vi "Maestro Ethernet Communication Example V1.00.00.vi"() -> ()   [LabVIEW 2021]
doc: "Data Client.vi displays data sent via TCP from Data Server. Once a TCP connection is open, the VI reads 4 bytes to determine the amount of data being sent. It then reads and charts that many bytes. If an error occurs or the stop button is pressed, it sends a \"Q\" to the Data Sender to notify it to quit."
panel:
  in  "file path":path
  in  "Save":bool
  in  "Connect":bool
  out "Readings":dbl format="%.6e"
  out "Maestro Online":bool
  in  "Send":bool
  in  "Command":string="*CAU"
  out "Waveform Chart":dbl(graph)=2.12187e-08
  out "Response":string="\r\n"
  in  "stop":bool
  in  "Address":string="192.168.0.44"
  in  "Port":i16=5000 min=1025 step=1
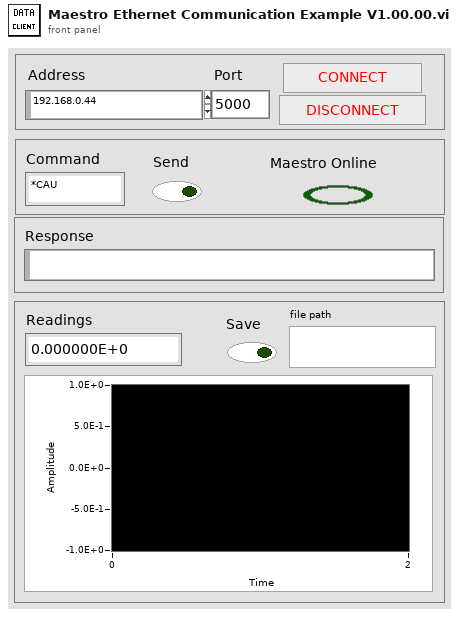
[diagram p1: front panel]
types:
  T1 = enum16{"Standard", "Buffered", "CRLF", "Immediate"}
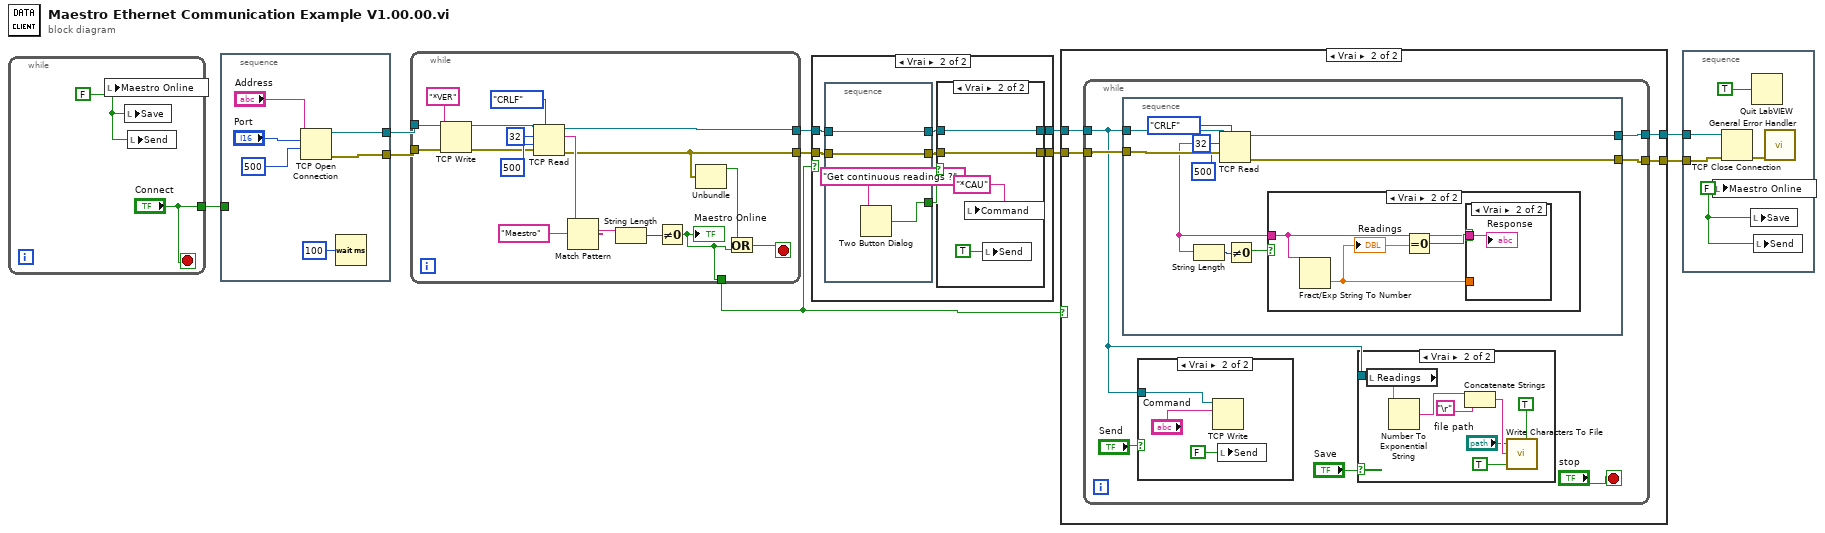
[diagram p0: block diagram]
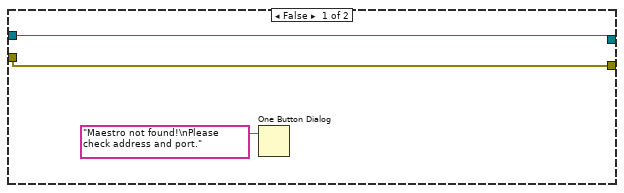
[diagram p4: hidden frame]
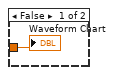
[diagram p7: hidden frame]
diagram:
  n1 = while {
    tunnel: ["Connect"] -> w2
    stop <- "Connect" stop-if-true
    w11 = FALSE ("Reception")
    n2 = local write "Maestro Online"(w11) -> ()
    n3 = local write "Save"(w11) -> ()
    n4 = local write "Send"(w11) -> ()
  }
  n5 = stacked-sequence {
    tunnel: [w16] -> w8
    tunnel: [w15] -> w7
    tunnel: w2 -> [_]
    frame #0 {
      n6 = TCP Open Connection(address="Address", remote port or service name="Port", timeout ms (60000)=500) -> (connection ID=w16:refnum<k5>, error out=w15:errorcluster)  [unwired: 2 in]
      n7 = Wait (ms)(milliseconds to wait=u32 100) -> ()  [unwired: 1 out]
    }
  }
  n8 = while {
    tunnel: [w35] -> w3
    tunnel: [w21] -> w4
    tunnel: w8 -> [w34]
    tunnel: w7 -> [w33]
    tunnel: [w19] -> w1
    stop <- w20 stop-if-true
    n9 = TCP Write(connection ID=w34, data in="*VER" ("string"), error in (no error)=w33) -> (connection ID out=w24:refnum<k5>, error out=w23:errorcluster)  [unwired: 1 in, 1 out]
    n10 = TCP Read(connection ID=w24, bytes to read=32, error in (no error)=w23, 7:T1."CRLF" ("mode (standard)"), 9:500 ("timeout ms (25000)")) -> (connection ID out=w35:refnum<k5>, data out=w29:string, error out=w21:errorcluster)
    n11 = Match Pattern(string=w29, regular expression="Maestro") -> (match substring=w26:string)  [unwired: 1 in, 3 out]
    n12 = String Length(string=w26) -> (length=w27:i32)
    n13 = Not Equal To 0?(x=w27) -> (x != 0?=w19:bool)
    "Maestro Online" <- w19
    n14 = Unbundle(w21) -> ("status"=w22:bool)  [unwired: 2 out]
    n15 = Or(x=w22, y=w19) -> (x .or. y?=w20:bool)
  }
  n16 = case shown="Vrai" w1 {
    tunnel: [w37 w44] -> w6
    tunnel: [w36 w43] -> w5
    tunnel: w4 -> [w37 w41]
    tunnel: w3 -> [w36 w40]
    frame False {
    }
    frame True {
      n17 = stacked-sequence {
        tunnel: [w48] -> w42
        tunnel: w41 -> [w47]
        tunnel: w40 -> [w46]
        tunnel: [w47] -> w39
        tunnel: [w46] -> w38
        frame #0 {
          n18 = Two Button Dialog(message="Get continuous readings ?") -> (T button?=w48:bool)  [unwired: 2 in]
        }
      }
      n19 = case shown="Vrai" w42 {
        tunnel: w39 -> [w49 w54]
        tunnel: [w49 w54] -> w44
        tunnel: [w50 w53] -> w43
        tunnel: w38 -> [w50 w53]
        frame False {
        }
        frame True {
          n20 = local write "Command"("*CAU" ("string")) -> ()
          n21 = local write "Send"(TRUE ("Send")) -> ()
        }
      }
    }
  }
  n22 = case shown="Vrai" w1 {
    tunnel: w5 -> [w57 w61]
    tunnel: w6 -> [w56 w60]
    tunnel: [w56 w59] -> w10
    tunnel: [w57 w58] -> w9
    frame False {
      n23 = One Button Dialog(message="Maestro not found!\nPlease check address and port.") -> ()  [unwired: 1 in, 1 out]
    }
    frame True {
      n24 = while {
        tunnel: w60 -> [w67]
        tunnel: w61 -> [w62]
        tunnel: [w66] -> w59
        tunnel: [w65] -> w58
        stop <- "stop" stop-if-true
        n25 = stacked-sequence {
          tunnel: w62 -> [w85]
          tunnel: w67 -> [w84]
          tunnel: [w83] -> w66
          tunnel: [w82] -> w65
          frame #0 {
            n26 = TCP Read(connection ID=w85, bytes to read=32, error in (no error)=w84, 7:T1."CRLF" ("mode (standard)"), 9:500 ("timeout ms (25000)")) -> (connection ID out=w82:refnum<k5>, data out=w76:string, error out=w83:errorcluster)
            n27 = String Length(string=w76) -> (length=w80:i32)
            n28 = Not Equal To 0?(x=w80) -> (x != 0?=w77:bool)
            n29 = case shown="Vrai" w77 {
              tunnel: w76 -> [_ w87]
              frame False {
              }
              frame True {
                n30 = Fract/Exp String To Number(string=w87) -> (number=w86:dbl)  [unwired: 3 in, 1 out]
                "Readings" <- w86
                n31 = Equal To 0?(x=w86) -> (x = 0?=w88:bool)
                n32 = case shown="Vrai" w88 {
                  tunnel: w87 -> [_ w90]
                  tunnel: w86 -> [w89 _]
                  frame False {
                    "Waveform Chart" <- w89
                  }
                  frame True {
                    "Response" <- w90
                  }
                }
              }
            }
          }
        }
        n33 = case shown="Vrai" "Send" {
          tunnel: w62 -> [_ w92]
          frame False {
          }
          frame True {
            n34 = TCP Write(connection ID=w92, data in="Command") -> ()  [unwired: 2 in, 3 out]
            n35 = local write "Send"(FALSE ("Send")) -> ()
          }
        }
        n36 = case shown="Vrai" "Save" {
          tunnel: w62 -> [_ _]
          frame False {
          }
          frame True {
            n37 = local read "Readings"() -> (w70:dbl)
            n38 = Number To Exponential String(number=w70) -> (E-format string=w71:string)  [unwired: 3 in]
            n39 = Concatenate Strings(w71, "\r") -> (w73:string)
            n40 = call <vilib>:"Write Characters To File.vi"("convert eol? (no:F)"=TRUE, "append to file? (new file:F)"=TRUE, "character string"=w73, "file path (dialog if empty)"="file path") -> ()  [unwired: 1 in, 1 out]
          }
        }
      }
    }
  }
  n41 = stacked-sequence {
    tunnel: w9 -> [w97]
    tunnel: w10 -> [w96]
    frame #0 {
      w95 = FALSE ("Reception")
      n42 = local write "Maestro Online"(w95) -> ()
      n43 = TCP Close Connection(connection ID=w97, error in (no error)=w96) -> (error out=w98:errorcluster)  [unwired: 1 in, 1 out]
      n44 = local write "Save"(w95) -> ()
      n45 = Quit LabVIEW(quit? (T)=TRUE) -> ()
      n46 = local write "Send"(w95) -> ()
      n47 = call <vilib>:"General Error Handler.vi"("error in (no error)"=w98) -> ()  [unwired: 10 in, 5 out]
    }
  }
